vi "Practica 12 - FormulaGeneral-SubVI.vi"(3 "C":dbl, 4 "B":dbl, 5 "A":dbl) -> (0 "RAIZ 2":dbl, 1 "RAIZ 1":dbl, 2 "TIPO DE RAIZ":string)   [LabVIEW 2023]
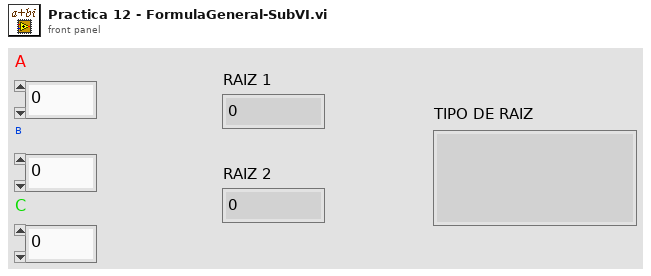
[diagram p1: front panel]
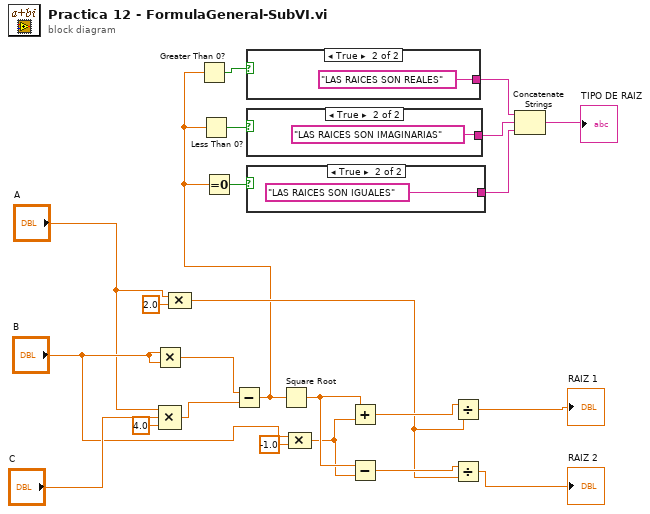
[diagram p0: block diagram]
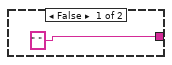
[diagram p2: hidden frame]
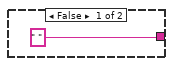
[diagram p3: hidden frame]
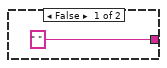
[diagram p4: hidden frame]
diagram:
  n1 = Multiply(x="B", y="B") -> (x*y=w23:dbl)
  n2 = Compound Arithmetic op=MULTIPLY("A", "C", 4.0 ("value")) -> (w22:dbl)
  n3 = Compound Arithmetic op=MULTIPLY("A", 2.0 ("value")) -> (w11:dbl)
  n4 = Subtract(x=w23, y=w22) -> (x-y=w1:dbl)
  n5 = Greater Than 0?(x=w1) -> (x > 0?=w10:bool)
  n6 = Less Than 0?(x=w1) -> (x < 0?=w9:bool)
  n7 = Equal To 0?(x=w1) -> (x = 0?=w2:bool)
  n8 = case shown="True" w10 {
    tunnel: [" " "LAS RAICES SON REALES"] -> w8
    frame False {
    }
    frame True {
    }
  }
  n9 = case shown="True" w9 {
    tunnel: [" " "LAS RAICES SON IMAGINARIAS"] -> w7
    frame False {
    }
    frame True {
    }
  }
  n10 = case shown="True" w2 {
    tunnel: [" " "LAS RAICES SON IGUALES"] -> w6
    frame False {
    }
    frame True {
    }
  }
  n11 = Square Root(x=w1) -> (sqrt(x)=w19:dbl)
  n12 = Compound Arithmetic op=MULTIPLY("B", -1.0 ("value")) -> (w18:dbl)
  n13 = Add(x=w19, y=w18) -> (x+y=w13:dbl)
  n14 = Subtract(x=w19, y=w18) -> (x-y=w12:dbl)
  n15 = Divide(x=w13, y=w11) -> (x/y=→"RAIZ 1":dbl)
  n16 = Divide(x=w12, y=w11) -> (x/y=→"RAIZ 2":dbl)
  n17 = Concatenate Strings(w8, w7, w6) -> (→"TIPO DE RAIZ":string)
